vi "Sensors_TC.vi"() -> ()   [LabVIEW 2018]
uses:
  <vilib>/DAQmx/read.llb/DAQmx Read (Analog 1D Wfm NChan NSamp).vi
  <vilib>/DAQmx/configure/timing.llb/DAQmx Timing (Sample Clock).vi
  <vilib>/DAQmx/configure/task.llb/DAQmx Configure Logging (TDMS).vi
  <vilib>/DAQmx/miscellaneous.llb/DAQmx Fill In Error Info.vi
panel:
  in  "Minimum time between \nreadings [ms]":u32
  in  "task/channels in":refnum<k21>="MyTemperatureTask"
  out "output cluster":cluster{"data":waveform(dbl)[]}={"data"=[{"t0"=timestamp(3619119511.6238775 s since 1904-01-01), "dt"=0.01111111, "Y"=[25.7405769878202], "attributes"=variant("NI_ChannelName"=variant(string "HVOF_T_W_in"), "NI_UnitDescription"=variant(string "Deg C"))}, {"t0"=timestamp(3619119511.6238775 s since 1904-01-01), "dt"=0.01111111, "Y"=[25.58620395475177], "attributes"=variant("NI_ChannelName"=variant(string "HVOF_T_W_out"), "NI_UnitDescription"=variant(string "Deg C"))}, {"t0"=timestamp(3619119511.625707 s since 1904-01-01), "dt"=0.01111111, "Y"=[24.28685238275812], "attributes"=variant("NI_ChannelName"=variant(string "Ambient Temp"), "NI_UnitDescription"=variant(string "Deg C"))}, {"t0"=timestamp(3619119511.625707 s since 1904-01-01), "dt"=0.01111111, "Y"=[2389.2012910256], "attributes"=variant("NI_ChannelName"=variant(string "SAMP_T_W_in2"), "NI_UnitDescription"=variant(string "Deg C"))}, {"t0"=timestamp(3619119511.6275373 s since 1904-01-01), "dt"=0.01111111, "Y"=[2388.788461544843], "attributes"=variant("NI_ChannelName"=variant(string "SAMP_T_W_out1"), "NI_UnitDescription"=variant(string "Deg C"))}, {"t0"=timestamp(3619119511.6275373 s since 1904-01-01), "dt"=0.01111111, "Y"=[2389.2012910256], "attributes"=variant("NI_ChannelName"=variant(string "SAMP_T_W_out2"), "NI_UnitDescription"=variant(string "Deg C"))}, {"t0"=timestamp(3619119511.6293674 s since 1904-01-01), "dt"=0.01111111, "Y"=[2389.082850090546], "attributes"=variant("NI_ChannelName"=variant(string "T10"), "NI_UnitDescription"=variant(string "Deg C"))}, {"t0"=timestamp(3619119511.6293674 s since 1904-01-01), "dt"=0.01111111, "Y"=[2388.6700338310975], "attributes"=variant("NI_ChannelName"=variant(string "T9"), "NI_UnitDescription"=variant(string "Deg C"))}, {"t0"=timestamp(3619119511.631197 s since 1904-01-01), "dt"=0.01111111, "Y"=[2388.788461544843], "attributes"=variant("NI_ChannelName"=variant(string "T7"), "NI_UnitDescription"=variant(string "Deg C"))}, {"t0"=timestamp(3619119511.631197 s since 1904-01-01), "dt"=0.01111111, "Y"=[2389.082850090546], "attributes"=variant("NI_ChannelName"=variant(string "T8"), "NI_UnitDescription"=variant(string "Deg C"))}]}
  in  "Samples per channel":i32=17
  in  "Sample Rate":dbl=90.0 format="%0.2f"
  out "File Size (Mb)":dbl=42.99609375
  out "Filepath":path=path "C:/Labview Test Data/2018-09-06/Sensors_TC (2)/RawDAQmx/Log_Sensors_TC (2)_0_DAQmx.tdms"
  in  "stop":bool
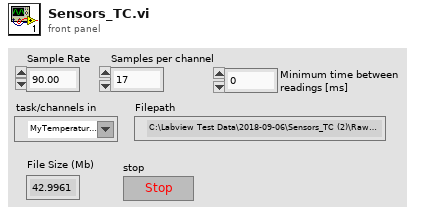
[diagram p1: front panel]
types:
  T1 = enum16{"open", "open or create", "create or replace", "create", "open (read-only)"}
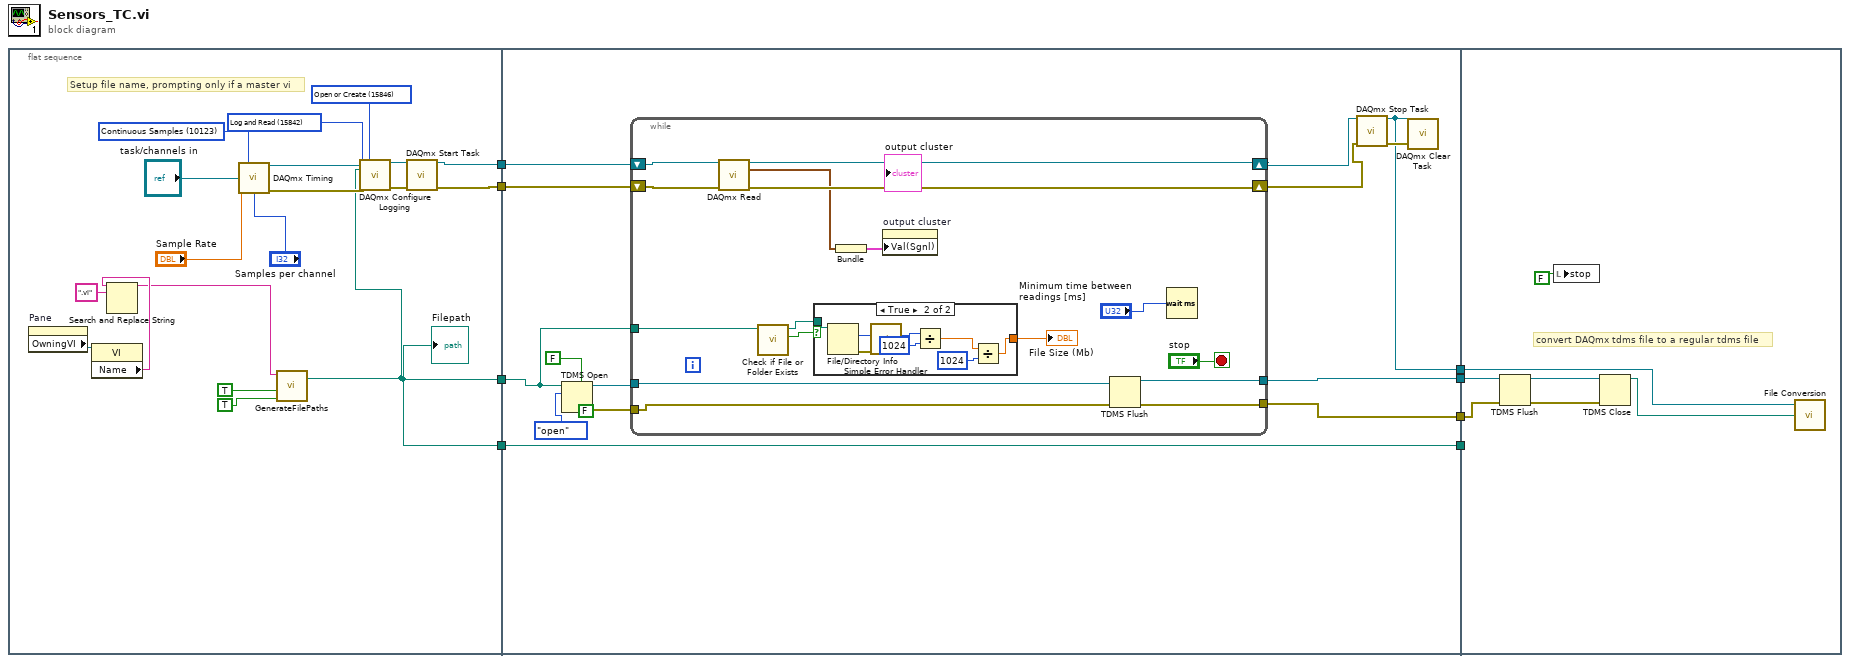
[diagram p0: block diagram]
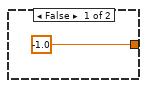
[diagram p2: hidden frame]
diagram:
  n1 = flat-sequence {
    tunnel: [w21] -> w8
    tunnel: [w26] -> w7
    tunnel: [w11] -> w6
    tunnel: [w11] -> w5
    tunnel: w8 -> [w41]
    tunnel: w7 -> [w40]
    tunnel: w6 -> [w36]
    tunnel: w5 -> [w32]
    tunnel: [w32] -> w4
    tunnel: [w31] -> w3
    tunnel: [w30] -> w2
    tunnel: [w28] -> w1
    tunnel: w4 -> [_]
    tunnel: w3 -> [w71]
    tunnel: w2 -> [w70]
    tunnel: w1 -> [w67]
    frame #0 {
      w14 = 10123 items=["Finite Samples"=10178, "Continuous Samples"=10123, "Hardware Timed Single Point"=12522] ("sample mode")
      w15 = 15842 items=["Off"=10231, "Log"=15844, "Log and Read"=15842] ("logging mode")
      w17 = 15846 items=["Open"=10437, "Open or Create"=15846, "Create or Replace"=15847, "Create"=15848] ("operation")
      # "Setup file name, prompting only if a master vi"
      n2 = property on="Pane" class="Pane"() -> ("OwningVI"=w27:refnum<vi>)  [unwired: 2 in, 2 out]
      n3 = property class="VI"(reference=w27) -> ("Name"=w10:string)  [unwired: 1 in, 2 out]
      n4 = Search and Replace String(input string=w10, search string=".vi") -> (result string=w9:string)  [unwired: 6 in, 3 out]
      n5 = call-poly <vilib>:"DAQmx Timing.vi"("task/channels in"="task/channels in", "sample mode"=w14, "samples per channel"="Samples per channel", "rate"="Sample Rate") -> ("task out"=w20:refnum<k21>, "error out"=w19:errorcluster)  [unwired: 10 in]
      n6 = call "GenerateFilePaths.vi"("Logfile?"=TRUE ("Instrument? (create folder)"), "DAQmx"=TRUE, "Device Name"=w9) -> ("Logfile Path"=w11:path)  [unwired: 1 in, 1 out]
      "Filepath" <- w11
      n7 = call-poly <vilib>:"DAQmx Configure Logging.vi"("task/channels in"=w20, "operation"=w17, "file path"=w11, "logging mode"=w15, "error in"=w19) -> ("task out"=w18:refnum<k21>, "error out"=w16:errorcluster)  [unwired: 9 in]
      n8 = call <vilib>:"DAQmx Start Task.vi"("task/channels in"=w18, "error in"=w16) -> ("task out"=w21:refnum<k21>, "error out"=w26:errorcluster)  [unwired: 12 in]
    }
    frame #1 {
      (unwired) FALSE ("create index file? (T)")
      n9 = TDMS Open(5:FALSE ("create index file? (T)"), 10:T1."open" ("operation (0:open)"), 11:w36) -> (0:w38:errorcluster, 3:w37:refnum<k34>)  [unwired: 4 in]
      n10 = while {
        shift-right: [w57] -> w33
        shift-left: w40 -> [w53]
        shift-right: [w54] -> w34
        shift-left: w41 -> [w55]
        tunnel: w37 -> [w49]
        tunnel: w38 -> [w48]
        tunnel: [w51] -> w31
        tunnel: [w50] -> w30
        tunnel: w36 -> [w42]
        stop <- "stop" stop-if-true
        n11 = call-poly <vilib>:"DAQmx Read.vi"("task/channels in"=w55, "error in"=w53) -> ("task out"=w54:refnum<k21>, "data"=w44:waveform(dbl)[], "error out"=w57:errorcluster)  [unwired: 11 in]
        n12 = call <vilib>:"Check if File or Folder Exists.vi"("path"=w42) -> ("file or folder exists?"=w46:bool, "dup path"=w47:path)  [unwired: 8 in, 1 out]
        n13 = case shown="True" w46 {
          tunnel: [-1.0 w59] -> w45
          tunnel: w47 -> [_ w62]
          frame False {
          }
          frame True {
            n14 = File/Directory Info(path=w62) -> (size=w65:i64, error out=w64:errorcluster)  [unwired: 1 in, 5 out]
            n15 = call <vilib>:"Simple Error Handler.vi"("error in (no error)"=w64) -> ()  [unwired: 1 in, 8 out]
            n16 = Divide(x=w65, y=i64 1024) -> (x/y=w60:dbl)
            n17 = Divide(x=w60, y=i64 1024) -> (x/y=w59:dbl)
          }
        }
        "File Size (Mb)" <- w45
        n18 = Bundle("data"=w44) -> (w43:cluster{"data":waveform(dbl)[]})  [unwired: 1 in]
        n19 = property on="output cluster" class="Clust (strict)"("Val(Sgnl)"=w43) -> ()  [unwired: 2 in, 2 out]
        n20 = TDMS Flush(4:w48, 7:w49) -> (0:w50:errorcluster, 3:w51:refnum<k34>)
        n21 = Wait (ms)(milliseconds to wait="Minimum time between \nreadings [ms]") -> ()  [unwired: 1 out]
      }
      n22 = call <vilib>:"DAQmx Stop Task.vi"("task/channels in"=w34, "error in"=w33) -> ("task out"=w28:refnum<k21>, "error out"=w35:errorcluster)  [unwired: 12 in]
      n23 = call <vilib>:"DAQmx Clear Task.vi"("task in"=w28, "error in"=w35) -> ()  [unwired: 13 in, 1 out]
    }
    frame #2 {
      # "convert DAQmx tdms file to a regular tdms file"
      n24 = TDMS Flush(4:w70, 7:w71) -> (0:w68:errorcluster, 3:w69:refnum<k34>)
      n25 = local write "stop"(FALSE ("stop")) -> ()
      n26 = TDMS Close(8:w68, 11:w69) -> (3:w66:path)  [unwired: 1 out]
      n27 = call "File Conversion.vi"("Initial File Path"=w66, "Task"=w67) -> ()  [unwired: 1 in]
    }
  }
